vi "ImageCounter.vi"(8 "error in (no error)":errorcluster, 11 "Image in":refnum<class "Image.lvclass">) -> (0 "error out":errorcluster, 2 "Image full":bool, 3 "Image out":refnum<class "Image.lvclass">, 4 "Frames grabbed":i32)   [LabVIEW 2012, in "Image.lvclass"]
uses:
  classes/Image.lvclass
  classes/Image.lvclass/Image.ctl
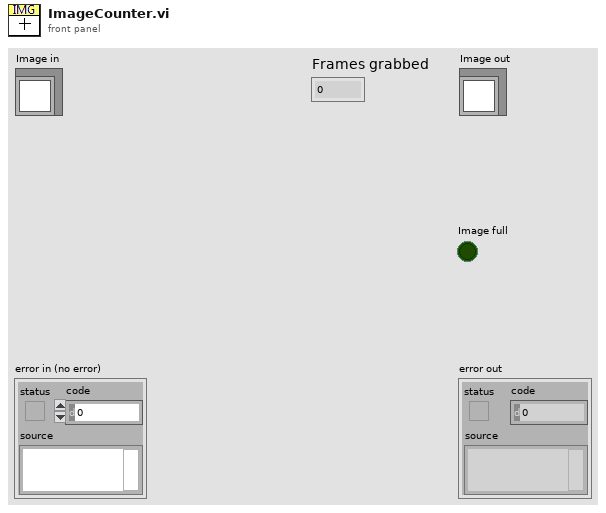
[diagram p1: front panel]
types:
  T1 = typedef "ScanMode.ctl" = enum16{"None", "Continuous", "Point Scan (CH3 cursor)", "Point Scan Move (CH3 cursor)", "Grab", "Grab Move Stage", "Grab Move Z-stage", "Cont. Move Z-stage", "Spec Move Stage", "Spec Move Cont", "Surf Calib"}
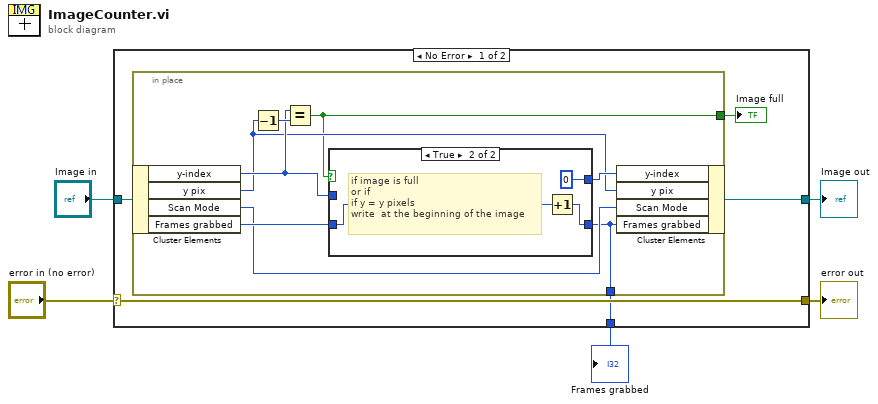
[diagram p0: block diagram]
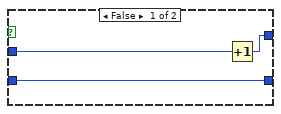
[diagram p2: hidden frame]
diagram:
  n1 = case shown="No Error" "error in (no error)" {
    selector: "error in (no error)" -> [w10 w26]
    tunnel: [w10 w26] -> w4
    tunnel: [w9 w25] -> w3
    tunnel: "Image in" -> [w7 w25]
    tunnel: [w6 _] -> w1
    frame No Error {
      n2 = in-place {
        in-place-border: [w14] -> w8
        in-place-border: [w11] -> w6
        n3 = in-place-cluster #1(w7) -> ("y-index"=w16:i32, "y pix"=w15:i32, "Scan Mode"=w12:T1, "Frames grabbed"=w13:i32)
        n4 = Decrement(x=w15) -> (x-1=w18:i32)
        n5 = Equal?(x=w16, y=w18) -> (x = y?=w14:bool)
        n6 = case shown="True" w14 {
          tunnel: w16 -> [w20 _]
          tunnel: [w21 0 ("t")] -> w17
          tunnel: [w19 w23] -> w11
          tunnel: w13 -> [w19 w22]
          frame False {
            n7 = Increment(x=w20) -> (x+1=w21:i32)
          }
          frame True {
            # "if image is full\nor if\nif y = y pixels\nwrite  at the beginning of the image"
            n8 = Increment(x=w22) -> (x+1=w23:i32)
          }
        }
        n9 = in-place-cluster #1("y-index"=w17, "y pix"=w15, "Scan Mode"=w12, "Frames grabbed"=w11) -> (w9:refnum<class "Image.lvclass">)
      }
      "Image full" <- w8
    }
    frame Error {
    }
  }
  "error out" <- w4
  "Image out" <- w3
  "Frames grabbed" <- w1
